vi "SliderColors.vi"() -> ()   [LabVIEW 2019]
panel:
  in  "Enter number":dbl
  out "Slider Control":dbl(slide)=5.0 scale=0.0..10.0
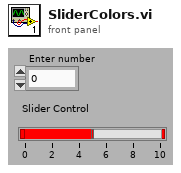
[diagram p1: front panel]
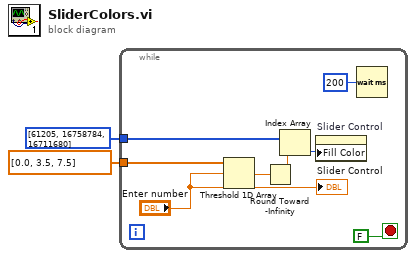
[diagram p0: block diagram]
diagram:
  n1 = while {
    tunnel: dbl[] [0.0, 3.5, 7.5] -> [w10]
    tunnel: u32[] [61205, 16758784, 16711680] -> [w9]
    stop <- FALSE ("stop") stop-if-true
    n2 = Threshold 1D Array(2:"Enter number", 3:w10) -> (0:w8:dbl)  [unwired: 1 in]
    n3 = Round Toward -Infinity(1:w8) -> (0:w6:dbl)
    n4 = Index Array(array=w9, index=w6) -> (element=w7:u32)
    n5 = property on="Slider Control" class="Slide (strict)"("Fill Color"=w7) -> ()  [unwired: 2 in, 2 out]
    n6 = Wait (ms)(milliseconds to wait=u32 200) -> ()  [unwired: 1 out]
    "Slider Control" <- "Enter number"
  }
